vi "Material-Line 1-CurandPlot.vi"(0 "Material-RunTest in":refnum<class "Material-RunTest.lvclass">, 5 "error in (no error)":errorcluster, 6 "Active Cursor Max":u32, 8 "Active Cursor Min":u32, 10 "Active Y Scale":i32, 12 "Active Plot":u32) -> (14 "Material-RunTest out":refnum<class "Material-RunTest.lvclass">, 19 "error out":errorcluster)   [LabVIEW 2013, in "Material-RunTest.lvclass"]
uses:
  Material-RunTest.lvclass
  Material-RunTest.lvclass/Material-RunTest.ctl
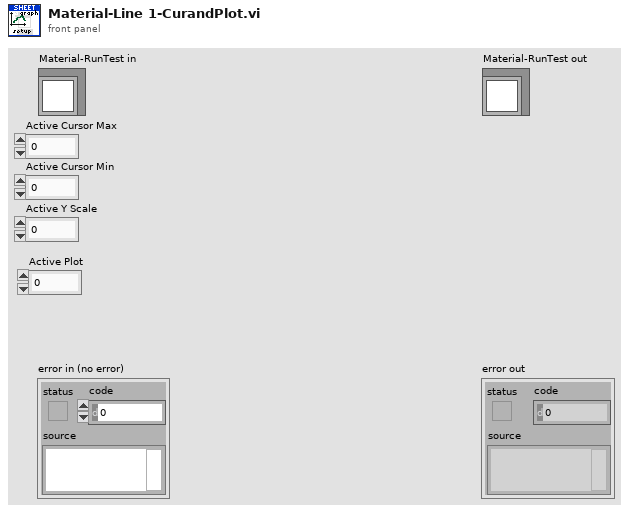
[diagram p1: front panel]
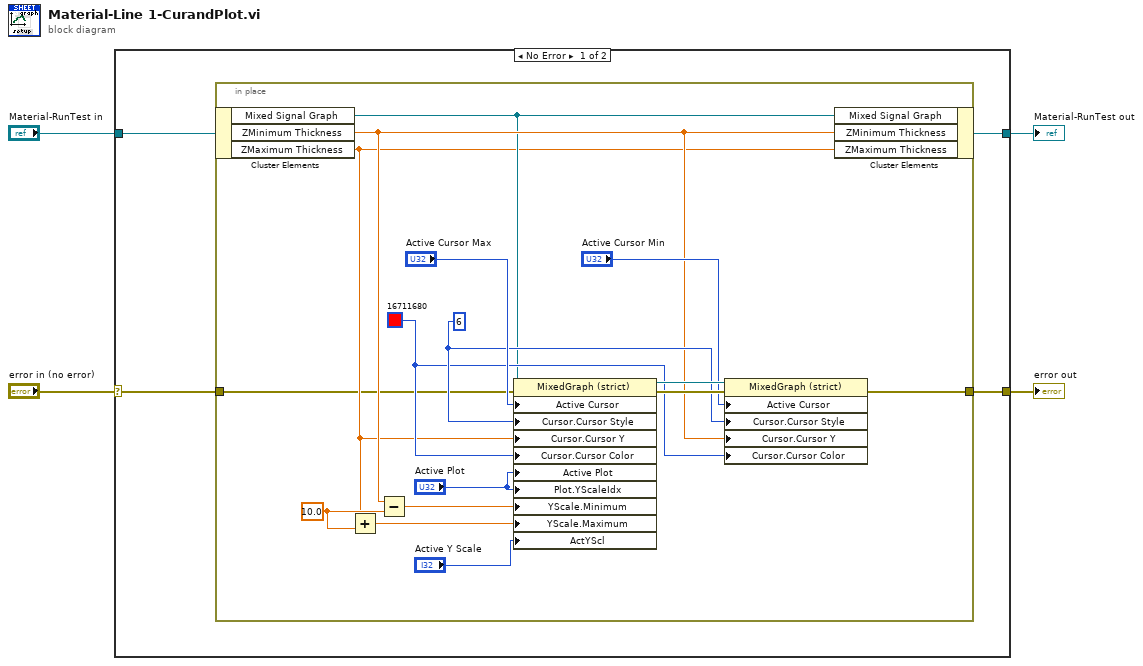
[diagram p0: block diagram]
diagram:
  n1 = case shown="No Error" "error in (no error)" {
    selector: "error in (no error)" -> [w6 w26]
    tunnel: [w5 w26] -> w3
    tunnel: [w7 w25] -> w1
    tunnel: "Material-RunTest in" -> [w8 w25]
    frame No Error {
      n2 = in-place {
        in-place-border: w6 -> [w10]
        in-place-border: [w9] -> w5
        w16 = u8 6 ("Cursor.Cursor Style")
        w15 = u32 16711680
        w22 = 10.0 ("y")
        n3 = in-place-cluster #1(w8) -> ("Mixed Signal Graph"=w12:refnum<vi>, "ZMinimum Thickness"=w13:dbl, "ZMaximum Thickness"=w11:dbl)
        n4 = Add(x=w11, y=w22) -> (x+y=w23:dbl)
        n5 = Subtract(x=w13, y=w22) -> (x-y=w24:dbl)
        n6 = property class="MixedGraph (strict)"(reference=w12, error in=w10, "Active Cursor"="Active Cursor Max", "Cursor.Cursor Style"=w16, "Cursor.Cursor Y"=w11, "Cursor.Cursor Color"=w15, "Active Plot"="Active Plot", "Plot.YScaleIdx"="Active Plot", "YScale.Minimum"=w24, "YScale.Maximum"=w23, "ActYScl"="Active Y Scale") -> (reference out=w18:refnum<vi>, error out=w19:errorcluster)
        n7 = property class="MixedGraph (strict)"(reference=w18, error in=w19, "Active Cursor"="Active Cursor Min", "Cursor.Cursor Style"=w16, "Cursor.Cursor Y"=w13, "Cursor.Cursor Color"=w15) -> (error out=w9:errorcluster)  [unwired: 1 out]
        n8 = in-place-cluster #1("Mixed Signal Graph"=w12, "ZMinimum Thickness"=w13, "ZMaximum Thickness"=w11) -> (w7:refnum<class "Material-RunTest.lvclass">)
      }
    }
    frame Error {
    }
  }
  "error out" <- w3
  "Material-RunTest out" <- w1
